vi "GetOutputPolarity.vi"(3 "error in (no error)":errorcluster, 4 "Channel (0: Channel 1)":u16(ring) items=["Channel 1", "Channel 2", "Channel 3", "Channel 4", "Channel 5", "Channel 6", "Channel 7", "Channel 8"], 5 "VISA resource name":refnum<visa-resource-name>) -> (0 "error out":errorcluster, 1 "Polarity":u8(ring) items=["Positive", "Negative"], 2 "VISA resource name out":refnum<visa-resource-name>)   [LabVIEW 2020, in "Active Technologies AWG3000.lvlib"]
uses:
  Active Technologies AWG3000.lvlib
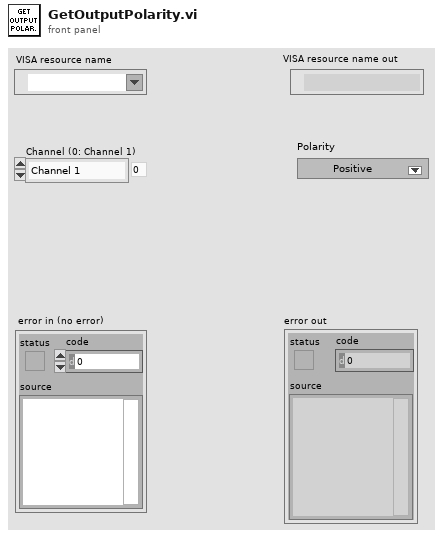
[diagram p1: front panel]
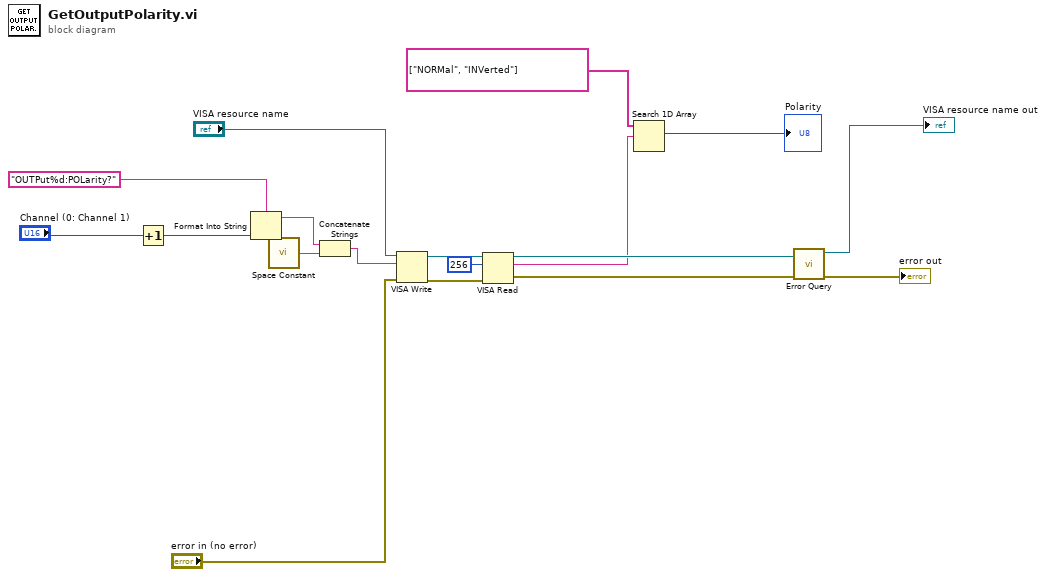
[diagram p0: block diagram]
diagram:
  n1 = Increment(x="Channel (0: Channel 1)") -> (x+1=w15:u16)
  n2 = Format Into String(format string="OUTPut%d:POLarity?" ("write buffer"), w15) -> (resulting string=w14:string)  [unwired: 2 in, 1 out]
  n3 = call <vilib>:"Space Constant.vi"() -> ("String"=w5:string)
  n4 = Concatenate Strings(w14, w5) -> (w13:string)
  n5 = VISA Write(VISA resource name="VISA resource name", write buffer=w13, error in (no error)="error in (no error)") -> (VISA resource name out=w12:refnum<visa-resource-name>, error out=w11:errorcluster)  [unwired: 1 out]
  n6 = VISA Read(VISA resource name=w12, byte count=u32 256, error in (no error)=w11) -> (VISA resource name out=w9:refnum<visa-resource-name>, read buffer=w3:string, error out=w8:errorcluster)  [unwired: 1 out]
  n7 = Search 1D Array(1D array=string[] ["NORMal", "INVerted"], element=w3) -> (index of element=→"Polarity":i32)  [unwired: 1 in]
  n8 = call "Error Query.vi"("error in (no error)"=w8, "VISA resource name"=w9) -> ("error out"=→"error out":errorcluster, "VISA resource name out"=→"VISA resource name out":refnum<visa-resource-name>)  [unwired: 6 in, 2 out]
